vi "TesterPresent.vi"(0 "reference in":refnum<class "UDS.lvclass">, 5 "error in (no error)":errorcluster) -> (14 "reference out":refnum<class "UDS.lvclass">, 19 "error out":errorcluster)   [LabVIEW 2020, in "UDS.lvclass"]
uses:
  UDS.lvclass
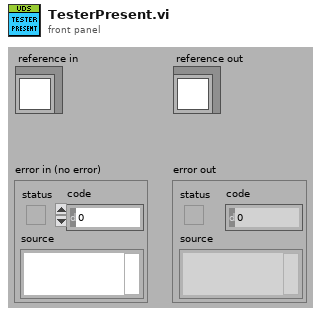
[diagram p1: front panel]
types:
  T1 = typedef "UDS.lvclass/ObjectAttributesRef.ctl" = refnum<data-value>
  T2 = typedef "UDS.lvclass/ObjectAttributes.ctl" = cluster{"MyAttribute":dbl, "UDSSetting":cluster{"InterfacName":string, "Baud Rate":u64, "FD Baud Rate":u64, "Transport Protocol":T3, "IO Mode":u32, "Max DLC":u16, "Transmit ID":u32, "Receive ID":u32, "Wait Time CF (STmin)":u32, "Fill Byte":u32}, "diag ref":T4}
  T3 = typedef "NI_Automotive Diagnostic Command Set.lvlib/Transport Protocol Selector.ctl" = enum16{"ISO TP - Normal Mode", "ISO TP - Mixed Mode", "VW TP 2.0", "Diagnostics on IP", "ISO TP LIN"}
  T4 = typedef "NI_Automotive Diagnostic Command Set.lvlib/Diag Reference.ctl" = cluster{"Diag CAN Handle":u32, "Transport Protocol":T3, "Receive Address Extension":u8, "Transmit Address Extension":u8, "Receive CAN Id":u32, "Transmit CAN Id":u32, "Log Frames ?":bool, "My TP Address":u8, "Other TP Address":u8, "T1":u16, "T2":u16, "T3":u16, "T4":u16, "Tx SN":u8, "Block Size":u8, "Rx SN":u8, "VW TP Initialized?":bool, "Tx block no":u8, "baud rate":u64, "Interface":string, "Channel Diag CAN Handle":u32, "UDP Connection ID":refnum<k16>, "TCP Connection ID":refnum<k5>, "Target IP Addr":u32, "Source Address":u16, "Target Address":u16, "Send Header NACK?":bool, "DLL Handle":u32, "NAD":u8, "Time Stamp read first":dbl, "Time Stamp read last":dbl, "Time Stamp write first":dbl, "Time Stamp write last":dbl, "Time Stamp write":dbl, "Time Stamp read":dbl, " I/O Mode":u32, "FD Baudrate":u64, "TX_DL":u16, "RX_DL":u16, "DoIP Protocol Version":T5, " Selected I/O Mode":u32, "TesterPresent Counter":u32, "TesterPresent Limit":u32, "TesterPresent Tick[ms]":i32, "TesterPresent RequireResponse?":bool, "TesterPresent Stored Ref?":bool, "TesterPresent Message":u8[], "TesterPresent Task Handle":i32, "TesterPresent Semaphore":T6, "Response Plausibility Check":u32, "Default Version?":bool, "Diagostic Globals":T7, "Session-based Properties?":bool}
  T5 = typedef "NI_Automotive Diagnostic Command Set.lvlib/DoIP Protocol Version.ctl" = u8
  T6 = typedef "Semaphore RefNum" = refnum<k1>
  T7 = typedef "NI_Automotive Diagnostic Command Set.lvlib/Diag Globals.ctl" = cluster{"Timeout FC (Bs)":u32, "Timeout CF (Cr)":u32, "Timeout Diag Command":u32, "Receive Block Size (BS)":u8, "Wait Time CF (STmin)":u8, "Max Waits (N_WFTmax)":u8, "Waits to Send (N_WAIT)":i32, "Time between Waits (TW)":u32, "Fill CAN Frames?":bool, "Fill Byte":u32, "Invalid Response as Error?":bool, "Max RspPending Count":u32, "VWTP Command Timeout":u32, "Transport Protocol":T3, "Diag CAN Handle":u32, "DLL Handle":u32, "Timeout RspPending":u32}
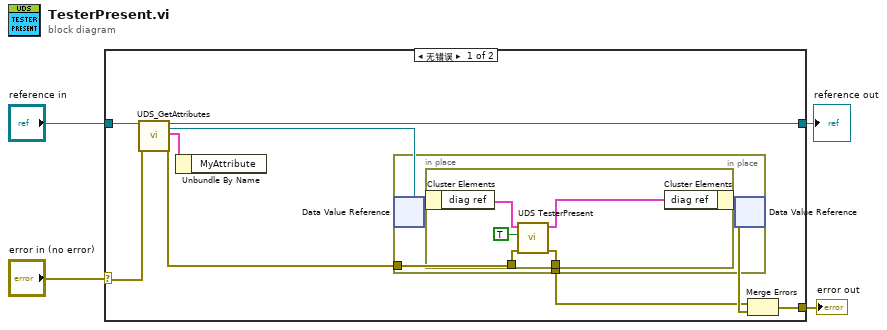
[diagram p0: block diagram]
diagram:
  n1 = case shown="无错误" "error in (no error)" {
    selector: "error in (no error)" -> [w10 w24]
    tunnel: [w13 w24] -> w3
    tunnel: [w11 w23] -> w1
    tunnel: "reference in" -> [w12 w23]
    frame No Error {
      n2 = call "UDS_GetAttributes.vi"("reference in"=w12, "error in (no error)"=w10) -> ("reference out"=w11:refnum<class "UDS.lvclass">, "attributes ref"=w6:T1, "attributes"=w8:T2, "error out"=w9:errorcluster)  [unwired: 14 in]
      n3 = Unbundle By Name(w8) -> ()  [unwired: 1 out]
      n4 = in-place {
        in-place-border: w9 -> [w15]
        in-place-border: [w14] -> w5
        n5 = in-place-dvr #1(w6) -> (w16:T2)  [unwired: 1 out]
        n6 = in-place {
          in-place-border: w15 -> [w19]
          in-place-border: [w18] -> w14
          n7 = in-place-cluster #2(w16) -> ("diag ref"=w22:T4)
          n8 = call <vilib>:"UDS TesterPresent.vi"("error in (no error)"=w19, "response required?"=TRUE, "diag ref in"=w22) -> ("error out"=w18:errorcluster, "diag ref out"=w21:T4)  [unwired: 7 out]
          n9 = in-place-cluster #2("diag ref"=w21) -> (w17:T2)
        }
        n10 = in-place-dvr #1(w17) -> (w7:errorcluster)  [unwired: 1 out]
      }
      n11 = Merge Errors(w5, w7) -> (w13:errorcluster)
    }
    frame Error {
    }
  }
  "error out" <- w3
  "reference out" <- w1
